vi "fix_wheel_turn.vi"(9 "wheel_fix":enum16{"l", "f", "r", "b"}(ring), 10 "Carzeta":dbl) -> ()   [LabVIEW 2017]
uses:
  Constant.vi
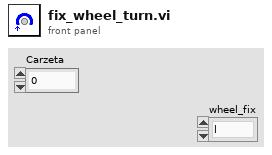
[diagram p1: front panel]
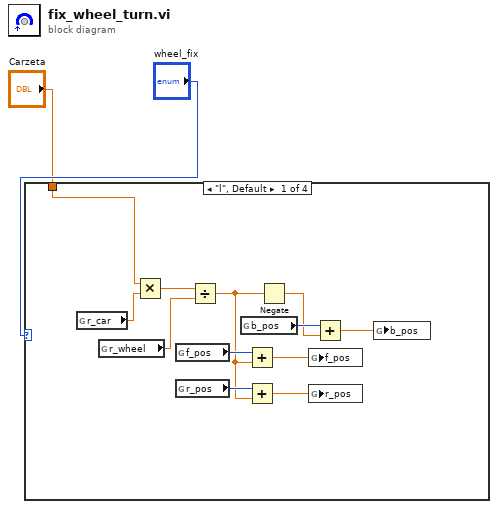
[diagram p0: block diagram]
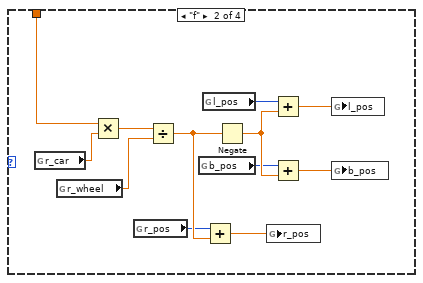
[diagram p2: hidden frame]
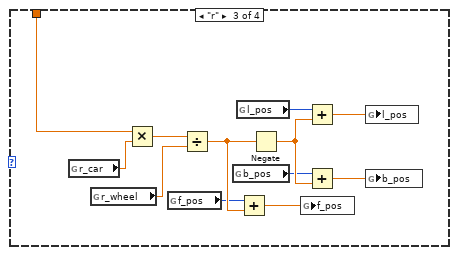
[diagram p3: hidden frame]
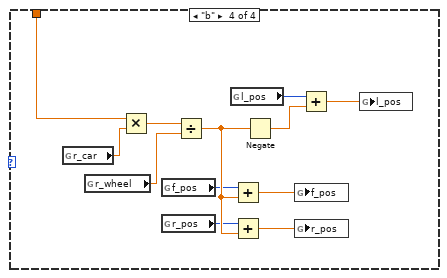
[diagram p4: hidden frame]
diagram:
  n1 = case shown="\"l\", Default" "wheel_fix" {
    tunnel: "Carzeta" -> [w3 w15 w27 w39]
    frame "l", Default {
      n2 = global read "Constant.vi" "r_car"() -> (w13:dbl)
      n3 = global read "Constant.vi" "r_wheel"() -> (w12:dbl)
      n4 = Multiply(x=w3, y=w13) -> (x*y=w14:dbl)
      n5 = global read "Constant.vi" "f_pos"() -> (w11:i32)
      n6 = global read "Constant.vi" "r_pos"() -> (w9:i32)
      n7 = Divide(x=w14, y=w12) -> (x/y=w4:dbl)
      n8 = global read "Constant.vi" "b_pos"() -> (w10:i32)
      n9 = Add(x=w11, y=w4) -> (x+y=w8:dbl)
      n10 = Add(x=w9, y=w4) -> (x+y=w6:dbl)
      n11 = Negate(x=w4) -> (-x=w5:dbl)
      n12 = global write "Constant.vi" "f_pos"(w8) -> ()
      n13 = global write "Constant.vi" "r_pos"(w6) -> ()
      n14 = Add(x=w10, y=w5) -> (x+y=w7:dbl)
      n15 = global write "Constant.vi" "b_pos"(w7) -> ()
    }
    frame "f" {
      n16 = global read "Constant.vi" "r_car"() -> (w17:dbl)
      n17 = global read "Constant.vi" "r_wheel"() -> (w18:dbl)
      n18 = Multiply(x=w15, y=w17) -> (x*y=w16:dbl)
      n19 = global read "Constant.vi" "r_pos"() -> (w21:i32)
      n20 = Divide(x=w16, y=w18) -> (x/y=w26:dbl)
      n21 = global read "Constant.vi" "b_pos"() -> (w20:i32)
      n22 = global read "Constant.vi" "l_pos"() -> (w19:i32)
      n23 = Add(x=w21, y=w26) -> (x+y=w24:dbl)
      n24 = Negate(x=w26) -> (-x=w25:dbl)
      n25 = global write "Constant.vi" "r_pos"(w24) -> ()
      n26 = Add(x=w19, y=w25) -> (x+y=w22:dbl)
      n27 = Add(x=w20, y=w25) -> (x+y=w23:dbl)
      n28 = global write "Constant.vi" "l_pos"(w22) -> ()
      n29 = global write "Constant.vi" "b_pos"(w23) -> ()
    }
    frame "r" {
      n30 = global read "Constant.vi" "r_car"() -> (w29:dbl)
      n31 = global read "Constant.vi" "r_wheel"() -> (w30:dbl)
      n32 = Multiply(x=w27, y=w29) -> (x*y=w28:dbl)
      n33 = global read "Constant.vi" "f_pos"() -> (w32:i32)
      n34 = Divide(x=w28, y=w30) -> (x/y=w38:dbl)
      n35 = global read "Constant.vi" "b_pos"() -> (w33:i32)
      n36 = global read "Constant.vi" "l_pos"() -> (w31:i32)
      n37 = Add(x=w32, y=w38) -> (x+y=w35:dbl)
      n38 = Negate(x=w38) -> (-x=w37:dbl)
      n39 = global write "Constant.vi" "f_pos"(w35) -> ()
      n40 = Add(x=w31, y=w37) -> (x+y=w34:dbl)
      n41 = Add(x=w33, y=w37) -> (x+y=w36:dbl)
      n42 = global write "Constant.vi" "l_pos"(w34) -> ()
      n43 = global write "Constant.vi" "b_pos"(w36) -> ()
    }
    frame "b" {
      n44 = global read "Constant.vi" "r_car"() -> (w41:dbl)
      n45 = global read "Constant.vi" "r_wheel"() -> (w42:dbl)
      n46 = Multiply(x=w39, y=w41) -> (x*y=w40:dbl)
      n47 = global read "Constant.vi" "f_pos"() -> (w44:i32)
      n48 = global read "Constant.vi" "r_pos"() -> (w45:i32)
      n49 = Divide(x=w40, y=w42) -> (x/y=w50:dbl)
      n50 = global read "Constant.vi" "l_pos"() -> (w43:i32)
      n51 = Add(x=w44, y=w50) -> (x+y=w47:dbl)
      n52 = Add(x=w45, y=w50) -> (x+y=w48:dbl)
      n53 = Negate(x=w50) -> (-x=w49:dbl)
      n54 = global write "Constant.vi" "f_pos"(w47) -> ()
      n55 = global write "Constant.vi" "r_pos"(w48) -> ()
      n56 = Add(x=w43, y=w49) -> (x+y=w46:dbl)
      n57 = global write "Constant.vi" "l_pos"(w46) -> ()
    }
  }
